vi "Init.vi"(8 "error in":errorcluster, 11 "object in":refnum<class "Scope PXI CFG.lvclass">) -> (0 "error out":errorcluster, 3 "object out":refnum<class "Scope PXI CFG.lvclass">)   [LabVIEW 2023, in "Scope.lvlib" / "Scope PXI.lvlib" / "Scope PXI CFG.lvclass"]
uses:
  Scope PXI CFG.lvclass
  Scope PXI CFG.lvclass/Scope PXI CFG.ctl
  Configuration Base/Configuration Base.lvclass
  7f301f3d-d01a-4c51-ac1c-d6c990f17446.vi
  D:/git/HAL/Configuration Base/Configuration Base.lvclass
  D:/git/HAL/Interfaces/IConfigure/IConfigure.lvclass
  D:/git/HAL/Scope PXI/Scope PXI CFG/Scope PXI CFG.lvclass
  <vilib>/ErrorRing/Error Ring.xnode
  <vilib>/Utility/error.llb/Error Cluster From Error Code.vi
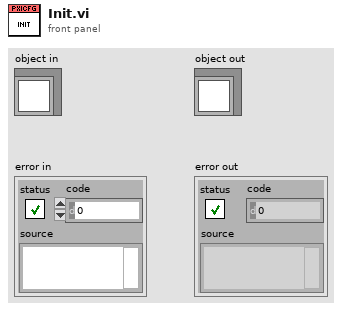
[diagram p1: front panel]
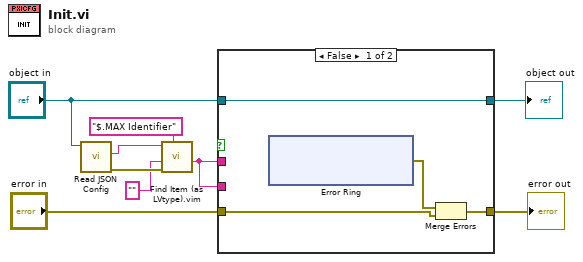
[diagram p0: block diagram]
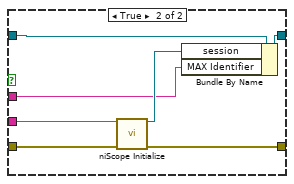
[diagram p2: hidden frame]
diagram:
  n1 = call "Read JSON Config.vi"("object in"="object in") -> ("error out"=w5:errorcluster, "<JSON>Config"=w6:string)  [unwired: 8 in, 1 out]
  n2 = call "Find Item (as LVtype).vim"("$Path or Item Name"="$.MAX Identifier", "error in (no error)"=w5, "Data Type and Default Value"="", "JSON"=w6) -> ("Data"=w1:string)  [unwired: 4 in, 3 out]
  n3 = case shown="False" {
    selector: _ -> [_ _]
    tunnel: "error in" -> [w11 w25]
    tunnel: [w13 w24] -> w8
    tunnel: [w10 w23] -> w7
    tunnel: "object in" -> [w10 w21]
    tunnel: w1 -> [_ w20]
    tunnel: w1 -> [_ w19]
    frame False {
      n4 = xnode "Error Ring"() -> ("error out"=w12:errorcluster)
      n5 = Merge Errors(w12, w11) -> (w13:errorcluster)
    }
    frame True {
      n6 = call <instrlib>:"niScope Initialize.vi"("resource name"=w20, "error in"=w25) -> ("instrument handle"=w22:refnum<k15>, "error out"=w24:errorcluster)  [unwired: 12 in]
      n7 = Bundle By Name(cluster=w21, "session"=w22, "MAX Identifier"=w19) -> (w23:refnum<class "Scope PXI CFG.lvclass">)
    }
  }
  "error out" <- w8
  "object out" <- w7
